vi "daq.io File Upload Download Example.vi"(8 "error in":errorcluster) -> (0 "error out":errorcluster)   [LabVIEW 2013, in "daqio minimal.lvlib"]
doc: "This examples demonstrates how to upload, download and delete files on the daq.io File store. Also, you can tie a file to a specific device so that it will show up on the device's page."
uses:
  daqio minimal.lvlib
  _typedefs/add-file-button.ctl
  _typedefs/download-button.ctl
  _typedefs/update-button.ctl
  _typedefs/exmpl_overlay_mask.ctl
  _typedefs/delete-button.ctl
  _typedefs/daqio-Credentials.ctl
  _typedefs/daqio-Type.ctl
  <vilib>/httpClient/ClientHandle.ctl
  <vilib>/Platform/browser.llb/Open URL in Default Browser (string).vi
  <vilib>/httpClient/LabVIEWHTTPClient.lvlib
panel:
  out "overlay mask":T1
  out "download succeeded":bool
  in  "folder to save the file to":path
  in  "Delete":T2
  in  "Refresh Files":T3
  in  "tie it to this device":bool
  in  "Your files on daq.io":i32(listbox)
  in  "Download File":T4
  in  "Upload File":T5
  in  "Stop":bool
  out "connected to daq.io":bool
  in  "Sign up link":bool caption="Boolean"
  out "Device Key":string
  in  "Log On":bool
  in  "User Name (your email)":string
  in  "Password":string
  # "Get your free account at daq.io first: sign up at"
  # "This Machine"
  # "(autogenerated in this example)"
  # "File Management"
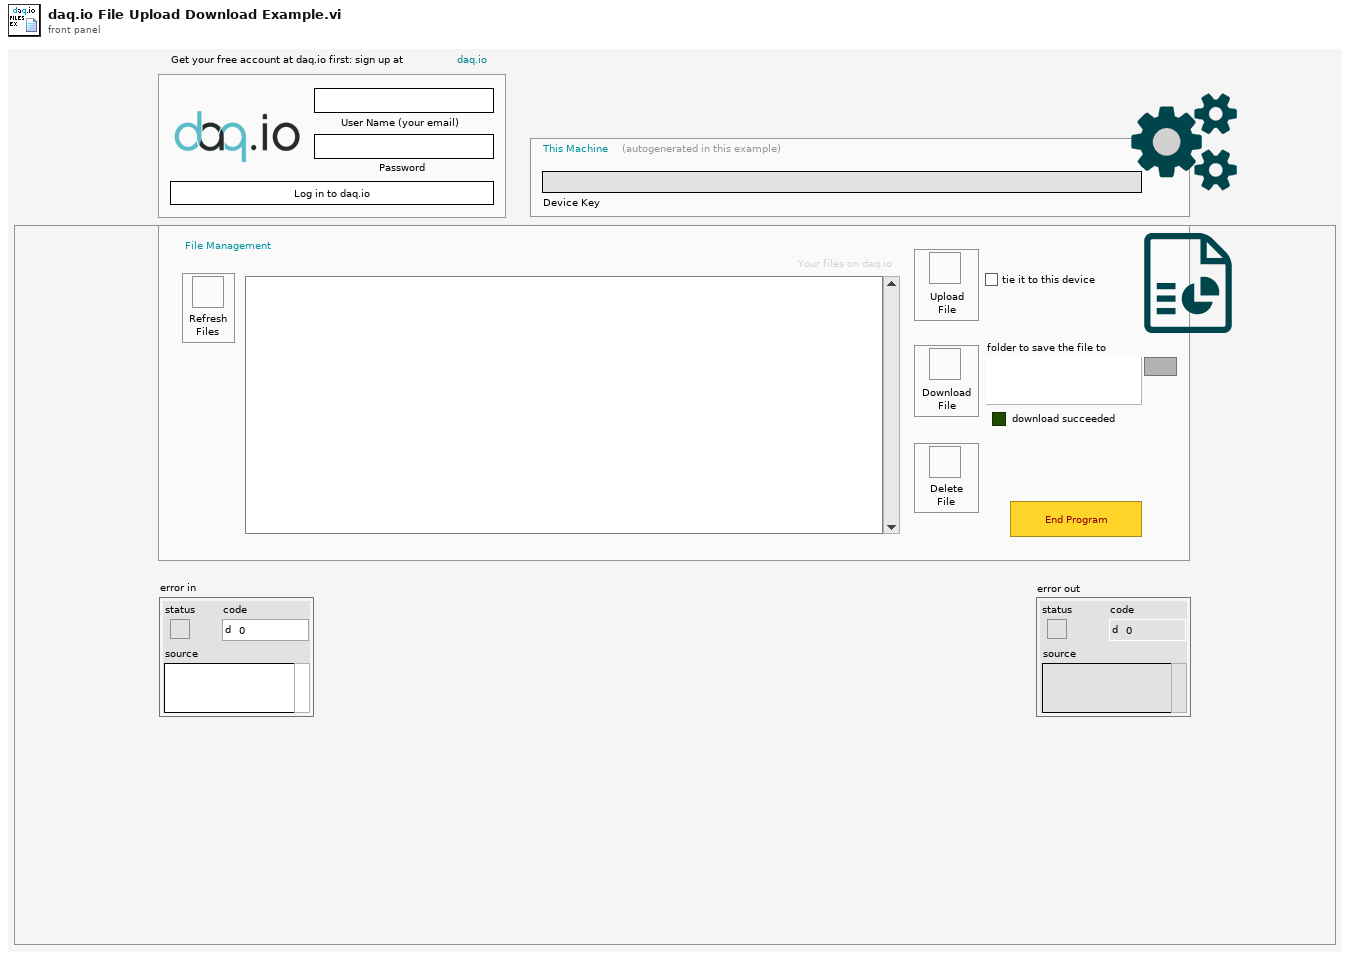
[diagram p1: front panel]
types:
  T1 = typedef "daqio minimal.lvlib/exmpl_overlay_mask.ctl" = bool
  T2 = typedef "daqio minimal.lvlib/delete-button.ctl" = bool
  T3 = typedef "daqio minimal.lvlib/update-button.ctl" = bool
  T4 = typedef "daqio minimal.lvlib/download-button.ctl" = bool
  T5 = typedef "daqio minimal.lvlib/add-file-button.ctl" = bool
  T6 = typedef "daqio minimal.lvlib/daqio-Credentials.ctl" = cluster{"User Name (email)":string, "Password":string}
  T7 = typedef "daqio minimal.lvlib/daqio-Type.ctl" = cluster{"daq.io ref":T8, "daq.io API Base":string, "Device Key":string, "Account ID":string, "online":bool, "SSL":bool}
  T8 = typedef "LabVIEWHTTPClient.lvlib/ClientHandle.ctl" = refnum<k1>
  T9 = typedef "daqio minimal.lvlib/daqio-File.ctl" = cluster{"id":string, "url":string, "file_type":string, "label":string, "original_file_name":string}
  T10 = cluster{"File Type":string, "label (File Name by default)":string, "File to be uploaded":path}
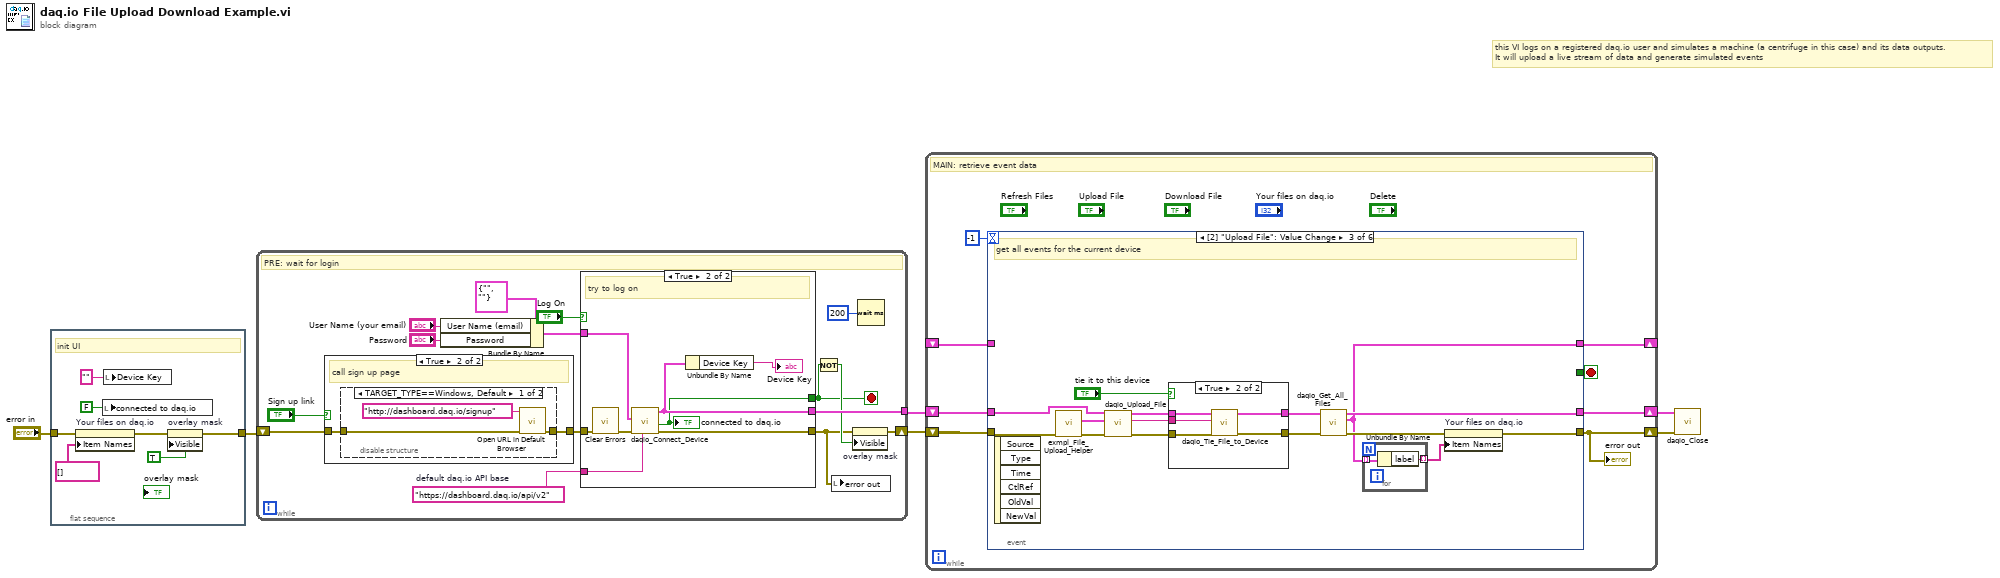
[diagram p0: block diagram]
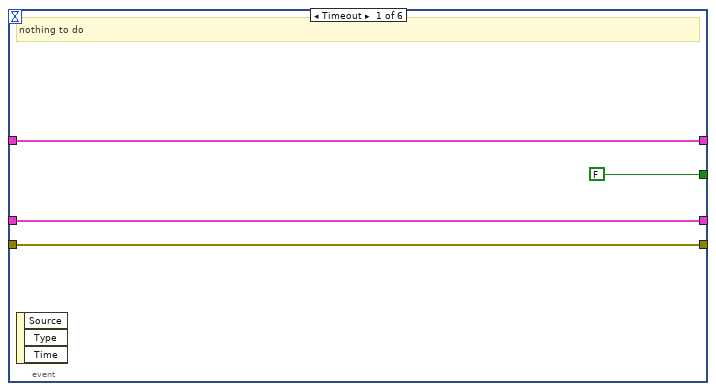
[diagram p2: hidden frame]
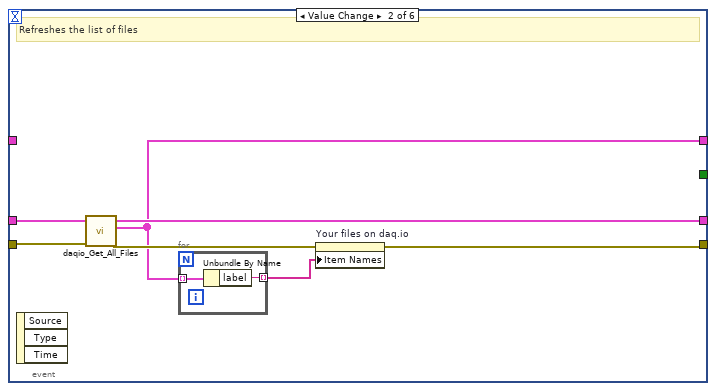
[diagram p3: hidden frame]
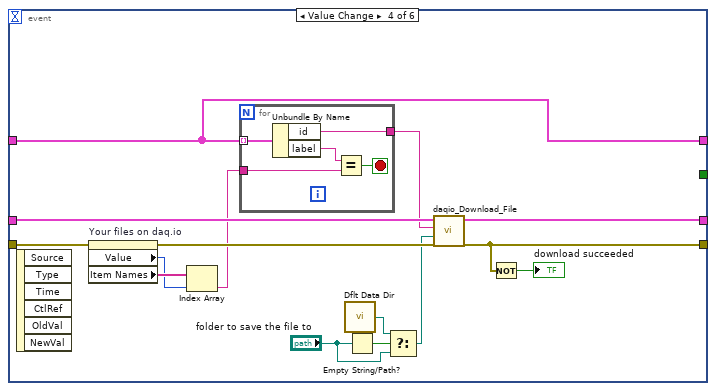
[diagram p5: hidden frame]
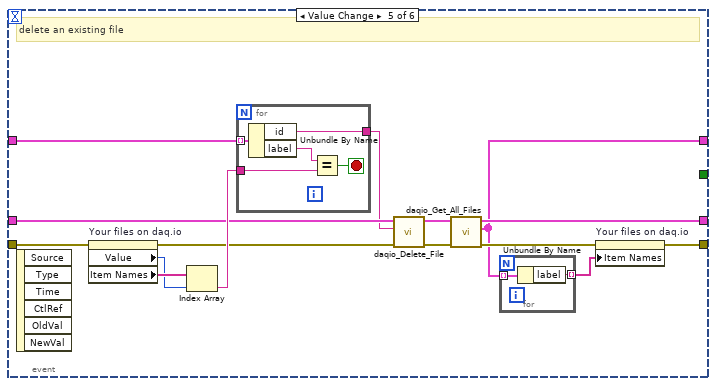
[diagram p6: hidden frame]
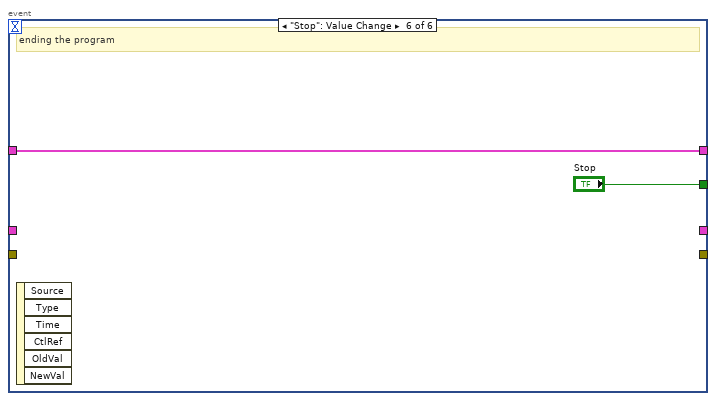
[diagram p7: hidden frame]
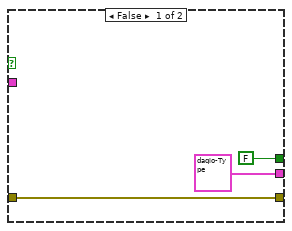
[diagram p10: hidden frame]
diagram:
  # "this VI logs on a registered daq.io user and simulates a machine (a centrifuge in this case) and its data outputs. \nIt will upload a live stream of data and generate simulated events"
  n1 = flat-sequence {
    tunnel: "error in" -> [w10]
    tunnel: [w9] -> w1
    frame #0 {
      # "init UI"
      n2 = property on="Your files on daq.io" class="LstBox (strict)"(error in=w10, "Item Names"=string[] []) -> (error out=w8:errorcluster)  [unwired: 1 in, 1 out]
      n3 = local write "connected to daq.io"(FALSE ("connected to daq.io")) -> ()
      n4 = local write "Device Key"("" ("log")) -> ()
      n5 = property on="overlay mask" class="Bool (strict)"(error in=w8, "Visible"=TRUE) -> (error out=w9:errorcluster)  [unwired: 1 in, 1 out]
    }
  }
  n6 = while {
    shift-right: [w14] -> w3
    shift-left: w1 -> [w21]
    tunnel: [w23] -> w4
    stop <- w16 stop-if-true
    w18 = "https://dashboard.daq.io/api/v2"  # default daq.io API base
    # "PRE: wait for login"
    n7 = case shown="True" "Sign up link" {
      tunnel: w21 -> [w29 w31]
      tunnel: [w29 w30] -> w20
      frame False {
      }
      frame True {
        # "call sign up page"
        n8 = disable-structure shown="TARGET_TYPE==Windows, Default" {
          disable-tunnel: w31 -> [w33 w35]
          disable-tunnel: [w32 w35] -> w30
          frame condition #0 (active) {
            n9 = call-poly <vilib>:"Open URL in Default Browser.vi"("error in (no error)"=w33, "URL"="http://dashboard.daq.io/signup") -> ("error out"=w32:errorcluster)  [unwired: 4 in, 1 out]
          }
          frame condition #1 {
          }
        }
      }
    }
    n10 = Bundle By Name(cluster=T6 {"User Name (email)"="", "Password"=""} ("daq.io Credentials"), "User Name (email)"="User Name (your email)", "Password"="Password") -> (w22:T6)
    n11 = case shown="True" "Log On" {
      tunnel: [T7 {"daq.io ref"=refnum, "daq.io API Base"="http://dashboard.daq.io/api/v1", "Device Key"="", "Account ID"="", "online"=FALSE, "SSL"=FALSE} ("daq.io type out") w42] -> w23
      tunnel: [w36 w46] -> w15
      tunnel: w20 -> [w36 w45]
      tunnel: w18 -> [_ w44]
      tunnel: w22 -> [_ w43]
      tunnel: [FALSE ("connected successfully?") w40] -> w16
      frame False {
      }
      frame True {
        # "try to log on"
        n12 = call <vilib>:"Clear Errors.vi"("error in (no error)"=w45) -> ("error out"=w39:errorcluster)  [unwired: 6 in]
        n13 = call "daqio_Connect_Device.vi"("daq.io API base"=w44, "error in (no error)"=w39, "Credentials"=w43) -> ("error out"=w46:errorcluster, "connected successfully?"=w40:bool, "daq.io type out"=w42:T7)  [unwired: 6 in]
        "connected to daq.io" <- w40
        n14 = Unbundle By Name(w42) -> ("Device Key"=→"Device Key":string)
      }
    }
    n15 = Not(x=w16) -> (.not. x?=w17:bool)
    n16 = local write "error out"(w15) -> ()
    n17 = property on="overlay mask" class="Bool (strict)"(error in=w15, "Visible"=w17) -> (error out=w14:errorcluster)  [unwired: 1 in, 1 out]
    n18 = Wait (ms)(milliseconds to wait=u32 200) -> ()  [unwired: 1 out]
  }
  n19 = while {
    shift-right: [w50] -> w6
    shift-left: w3 -> [w53]
    shift-right: [w52] -> w2
    shift-left: w4 -> [w54]
    shift-right: [w49] -> _
    shift-left: _ -> [w48]
    stop <- w51 stop-if-true
    # "MAIN: retrieve event data"
    n20 = event shown="[2] \"Upload File\": Value Change" {
      selector: _ -> [_ _ _ _ _ _]
      dyn-events: _ -> [_ _ _ _ _ _]
      timeout: -1 -> [_ _ _ _ _ _]
      tunnel: w54 -> [w57 w65 w81 w106 w120 _]
      tunnel: w53 -> [w56 w64 w69 w105 w125 _]
      tunnel: [w57 w60 w72 w95 w114 _] -> w52
      tunnel: [w56 w61 w74 w94 w113 _] -> w50
      tunnel: [FALSE ("Stop") _ _ _ _ "Stop"] -> w51
      tunnel: [w55 w59 w70 w92 w112 w134] -> w49
      tunnel: w48 -> [w55 _ _ w92 w126 w134]
      event Timeout {
        # "nothing to do"
        n21 = event-data() -> ()  [unwired: 1 in, 3 out]
      }
      event Value Change {
        # "Refreshes the list of files"
        n22 = event-data() -> ()  [unwired: 1 in, 3 out]
        n23 = call "daqio_Get_All_Files.vi"("error in (no error)"=w64, "daq.io type in"=w65) -> ("error out"=w62:errorcluster, "Existing Files"=w59:T9[], "daq.io type out"=w60:T7)  [unwired: 7 in]
        n24 = for {
          tunnel: w59 -> [w67] mode=indexing
          tunnel: [w66] -> w63 mode=indexing
          n25 = Unbundle By Name(w67) -> ("label"=w66:string)
        }
        n26 = property on="Your files on daq.io" class="LstBox (strict)"(error in=w62, "Item Names"=w63) -> (error out=w61:errorcluster)  [unwired: 1 in, 1 out]
      }
      event Value Change {
        # "get all events for the current device"
        n27 = event-data() -> ()  [unwired: 1 in, 6 out]
        n28 = call "exmpl_File_Upload_Helper.vi"("error in"=w69) -> ("error out"=w68:errorcluster, "output cluster"=w77:T10)  [unwired: 9 in]
        n29 = call "daqio_Upload_File.vi"("error in (no error)"=w68, "File to upload"=w77, "daq.io type in"=w81) -> ("error out"=w79:errorcluster, "asset ID"=w78:string, "daq.io type out"=w80:T7)  [unwired: 6 in]
        n30 = case shown="True" "tie it to this device" {
          tunnel: w80 -> [w86 w91]
          tunnel: w79 -> [w85 w90]
          tunnel: [w85 w89] -> w75
          tunnel: [w86 w88] -> w76
          tunnel: w78 -> [_ w87]
          frame False {
          }
          frame True {
            n31 = call "daqio_Tie_File_to_Device.vi"("error in (no error)"=w90, "file ID"=w87, "daq.io type in"=w91) -> ("error out"=w89:errorcluster, "daq.io type out"=w88:T7)  [unwired: 7 in]
          }
        }
        n32 = call "daqio_Get_All_Files.vi"("error in (no error)"=w75, "daq.io type in"=w76) -> ("error out"=w73:errorcluster, "Existing Files"=w70:T9[], "daq.io type out"=w72:T7)  [unwired: 7 in]
        n33 = for {
          tunnel: w70 -> [w84] mode=indexing
          tunnel: [w83] -> w71 mode=indexing
          n34 = Unbundle By Name(w84) -> ("label"=w83:string)
        }
        n35 = property on="Your files on daq.io" class="LstBox (strict)"(error in=w73, "Item Names"=w71) -> (error out=w74:errorcluster)  [unwired: 1 in, 1 out]
      }
      event Value Change {
        n36 = event-data() -> ()  [unwired: 1 in, 6 out]
        n37 = property on="Your files on daq.io" class="LstBox (strict)"(error in=w105) -> (error out=w104:errorcluster, "Value"=w102:i32, "Item Names"=w103:string[])  [unwired: 1 in, 1 out]
        n38 = Index Array(array=w103, index=w102) -> (element=w101:string)
        n39 = for {
          tunnel: w92 -> [w111] mode=indexing
          tunnel: w101 -> [w109]
          tunnel: [w107] -> w100
          stop <- w108 stop-if-true
          n40 = Unbundle By Name(w111) -> ("id"=w107:string, "label"=w110:string)
          n41 = Equal?(x=w110, y=w109) -> (x = y?=w108:bool)
        }
        n42 = call <vilib>:"Dflt Data Dir.vi"() -> ("App:Default Data Directory"=w98:path)
        n43 = Empty String/Path?(string/path="folder to save the file to") -> (empty?=w99:bool)
        n44 = Select(t=w98, s=w99, f="folder to save the file to") -> (s? t:f=w96:path)
        n45 = call "daqio_Download_File.vi"("error in (no error)"=w104, "folder to save the file to"=w96, "daq.io file ID"=w100, "daq.io type in"=w106) -> ("error out"=w94:errorcluster, "daq.io type out"=w95:T7)  [unwired: 6 in]
        n46 = Not(x=w94) -> (.not. x?=→"download succeeded":bool)
      }
      event Value Change {
        # "delete an existing file"
        n47 = event-data() -> ()  [unwired: 1 in, 6 out]
        n48 = property on="Your files on daq.io" class="LstBox (strict)"(error in=w125) -> (error out=w121:errorcluster, "Value"=w123:i32, "Item Names"=w124:string[])  [unwired: 1 in, 1 out]
        n49 = Index Array(array=w124, index=w123) -> (element=w122:string)
        n50 = for {
          tunnel: w126 -> [w133] mode=indexing
          tunnel: w122 -> [w131]
          tunnel: [w129] -> w119
          stop <- w130 stop-if-true
          n51 = Unbundle By Name(w133) -> ("id"=w129:string, "label"=w132:string)
          n52 = Equal?(x=w132, y=w131) -> (x = y?=w130:bool)
        }
        n53 = call "daqio_Delete_File.vi"("error in (no error)"=w121, "daq.io file ID"=w119, "daq.io type in"=w120) -> ("error out"=w116:errorcluster, "daq.io type out"=w115:T7)  [unwired: 7 in]
        n54 = call "daqio_Get_All_Files.vi"("error in (no error)"=w116, "daq.io type in"=w115) -> ("error out"=w118:errorcluster, "Existing Files"=w112:T9[], "daq.io type out"=w114:T7)  [unwired: 7 in]
        n55 = for {
          tunnel: w112 -> [w128] mode=indexing
          tunnel: [w127] -> w117 mode=indexing
          n56 = Unbundle By Name(w128) -> ("label"=w127:string)
        }
        n57 = property on="Your files on daq.io" class="LstBox (strict)"(error in=w118, "Item Names"=w117) -> (error out=w113:errorcluster)  [unwired: 1 in, 1 out]
      }
      event "Stop": Value Change {
        # "ending the program"
        n58 = event-data() -> ()  [unwired: 1 in, 6 out]
      }
    }
    "error out" <- w50
  }
  n59 = call "daqio_Close.vi"("error in (no error)"=w6, "daq.io type"=w2) -> ()  [unwired: 9 in, 1 out]
